vi "test Duplicate.vi"(8 "error in (no error)":errorcluster, 11 "TestCase In":refnum<class "Data Manipulation Tests.lvclass">) -> (0 "error out":errorcluster, 3 "TestCase Out":refnum<class "Data Manipulation Tests.lvclass">)   [LabVIEW 2017, in "Memory Manager Tests.lvlib" / "Data Manipulation Tests.lvclass"]
uses:
  Data Manipulation Tests.lvclass
  Source/Classes/Pointer/Write 1D I32.vi
  <vilib>/addons/_JKI Toolkits/VI Tester/TestCase.llb/TestCase.lvclass
  Source/Classes/Pointer/Pointer.lvclass
  C:/Program Files (x86)/National Instruments/LabVIEW 2017/vi.lib/addons/_JKI Toolkits/VI Tester/TestCase.llb/TestCase.lvclass
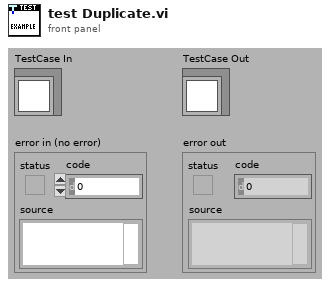
[diagram p1: front panel]
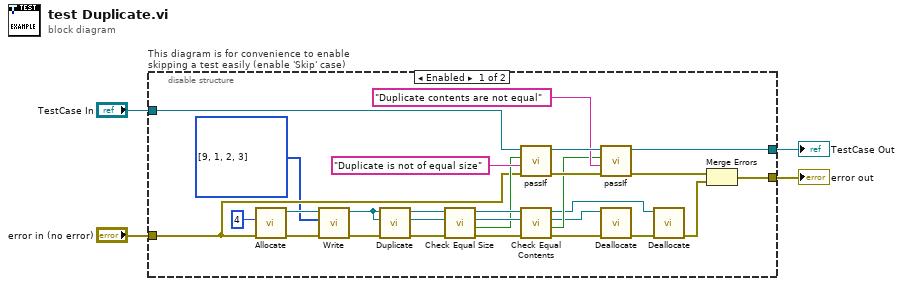
[diagram p0: block diagram]
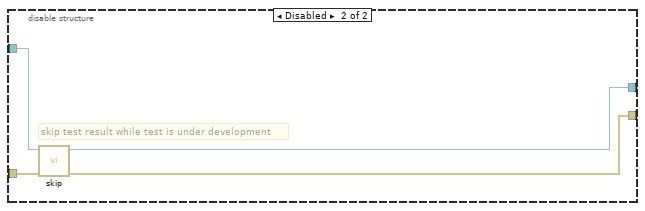
[diagram p2: hidden frame]
diagram:
  n1 = disable-structure "This diagram is for convenience to enable skipping a test easily (enable 'Skip' case)" shown="Enabled" {
    disable-tunnel: "TestCase In" -> [w30 w36]
    disable-tunnel: [w27 w34] -> w1
    disable-tunnel: [w13 w35] -> w3
    disable-tunnel: "error in (no error)" -> [w11 w33]
    frame Enabled {
      n2 = call "Allocate.vi"("error in (no error)"=w11, "size"=u64 4 ("count (1)")) -> ("error out"=w16:errorcluster, "Pointer out"=w32:refnum<class "Pointer.lvclass">)  [unwired: 8 in]
      n3 = call-poly "Write.vi"("error in (no error)"=w16, "buffer in"=i32[] [9, 1, 2, 3] ("count (1)"), "Pointer in"=w32) -> ("error out"=w15:errorcluster, "Pointer out"=w5:refnum<class "Pointer.lvclass">)  [unwired: 5 in, 2 out]
      n4 = call "Duplicate.vi"("error in (no error)"=w15, "new Pointer type"=w5, "Pointer in"=w5) -> ("error out"=w23:errorcluster, "new Pointer"=w20:refnum<class "Pointer.lvclass">, "Pointer out"=w24:refnum<class "Pointer.lvclass">)  [unwired: 6 in]
      n5 = call "Check Equal Size.vi"("error in (no error)"=w23, "Pointer y"=w20, "Pointer x"=w24) -> ("error out"=w21:errorcluster, "equal size?"=w18:bool, "Pointer y"=w19:refnum<class "Pointer.lvclass">, "Pointer x"=w22:refnum<class "Pointer.lvclass">)  [unwired: 5 in]
      n6 = call-dynamic "passIf.vi"("error in (no error)"=w11, "message (\"\")"="Duplicate is not of equal size" ("message (\"\")"), "pass"=w18, "TestCase in"=w30) -> ("error out"=w31:errorcluster, "TestCase out"=w28:refnum<class "Data Manipulation Tests.lvclass">)  [unwired: 6 in]
      n7 = call "Check Equal Contents.vi"("error in (no error)"=w21, "Pointer y"=w19, "Pointer x"=w22) -> ("error out"=w12:errorcluster, "equal contents?"=w17:bool, "Pointer y"=w8:refnum<class "Pointer.lvclass">, "Pointer x"=w7:refnum<class "Pointer.lvclass">)  [unwired: 5 in]
      n8 = call-dynamic "passIf.vi"("error in (no error)"=w31, "message (\"\")"="Duplicate contents are not equal" ("message (\"\")"), "pass"=w17, "TestCase in"=w28) -> ("error out"=w29:errorcluster, "TestCase out"=w27:refnum<class "Data Manipulation Tests.lvclass">)  [unwired: 6 in]
      n9 = call "Deallocate.vi"("error in (no error)"=w12, "Pointer"=w8) -> ("error out"=w10:errorcluster)  [unwired: 8 in, 1 out]
      n10 = call "Deallocate.vi"("error in (no error)"=w10, "Pointer"=w7) -> ("error out"=w9:errorcluster)  [unwired: 8 in, 1 out]
      n11 = Merge Errors(w29, w9) -> (w13:errorcluster)
    }
    frame Disabled {
      # "skip test result while test is under development"
      n12 = call <vilib>:"skip.vi"("error in (no error)"=w33, "TestCase in"=w36) -> ("error out"=w35:errorcluster, "TestCase out"=w34:refnum<class "Data Manipulation Tests.lvclass">)  [unwired: 8 in]
    }
  }
  "error out" <- w3
  "TestCase Out" <- w1
